vi "Acq-module.vi"(7 "IntermediateFIFO":refnum<k21>="FIFO0", 8 "NumChannels":T1, 9 "SamplingRate0":u16=10000, 11 "Cluster in":T3) -> (3 "cluster out":T4)   [LabVIEW 2013]
uses:
  ctl.ctl
  N Channels.ctl
  <vilib>/rvi/DataTransferAndStorage/Container/Common/niFpgaContainerExecOnDevCompGetState.vi
  <vilib>/rvi/FIFO/Fifo_Resource/nirvififoEmulationWriteFpgaImpl.vi
  <vilib>/rvi/DataTransferAndStorage/Container/Common/niFpgaContainerGetUniqueNameForEmu.vi
  <vilib>/rvi/interface/RandomDataEmulation/nirviRandomDataFPGAFIFO.vi
  <vilib>/rvi/interface/RandomDataEmulation/niFpgaRandomDataHandleErrors.vi
  <vilib>/rvi/eio/common/nirviEmuReportErrorAndStop.vi
  GlobalReg.vi
  <vilib>/rvi/DataTransferAndStorage/Container/XNode/niFpgaContainer.xnode
  <vilib>/rvi/FIFO/Fifo_Resource/niFpgaFifoEmulationRefIn.vi
panel:
  out "Analog Out Cluster":T2
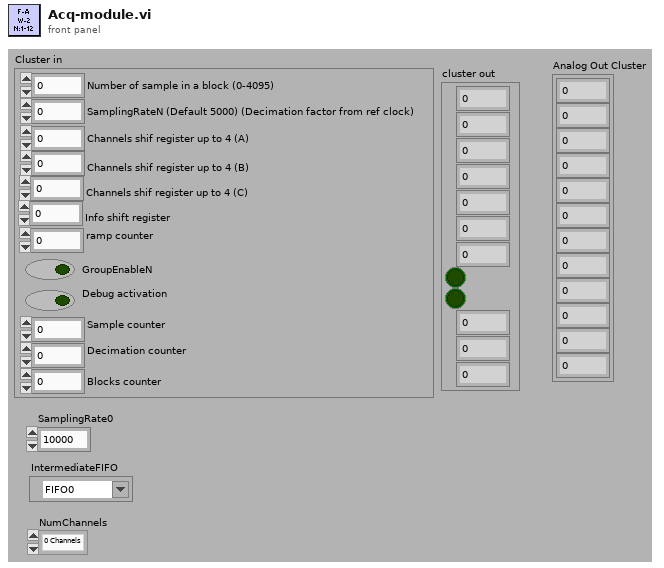
[diagram p1: front panel]
types:
  T1 = typedef "N Channels.ctl" = enum16{"0 Channels", "1 Channels", "2 Channels", "3 Channels", "4 Channels", "5 Channels", "6 Channels", "7 Channels", "8 Channels", "9 Channels", "10 Channels", "11 Channels", "12 Channels"}
  T2 = cluster{i16, i16, i16, i16, i16, i16, i16, i16, i16, i16, i16, i16}
  T3 = typedef "ctl.ctl" = cluster{"Number of sample in a block (0-4095)":u16, "SamplingRateN (Default 5000) (Decimation factor from ref clock)":u16, "Channels shif register up to 4 (A) ":u64, "Channels shif register up to 4 (B) ":u64, "Channels shif register up to 4 (C) ":u64, "Info shift register":u64, "ramp counter":i16, "GroupEnableN":bool, "Debug activation":bool, "Sample counter ":u64, "Decimation counter":u16, "Blocks counter":u16}
  T4 = cluster{u16, u16, u64, u64, u64, u64, i16, bool, bool, u64, u16, u16}
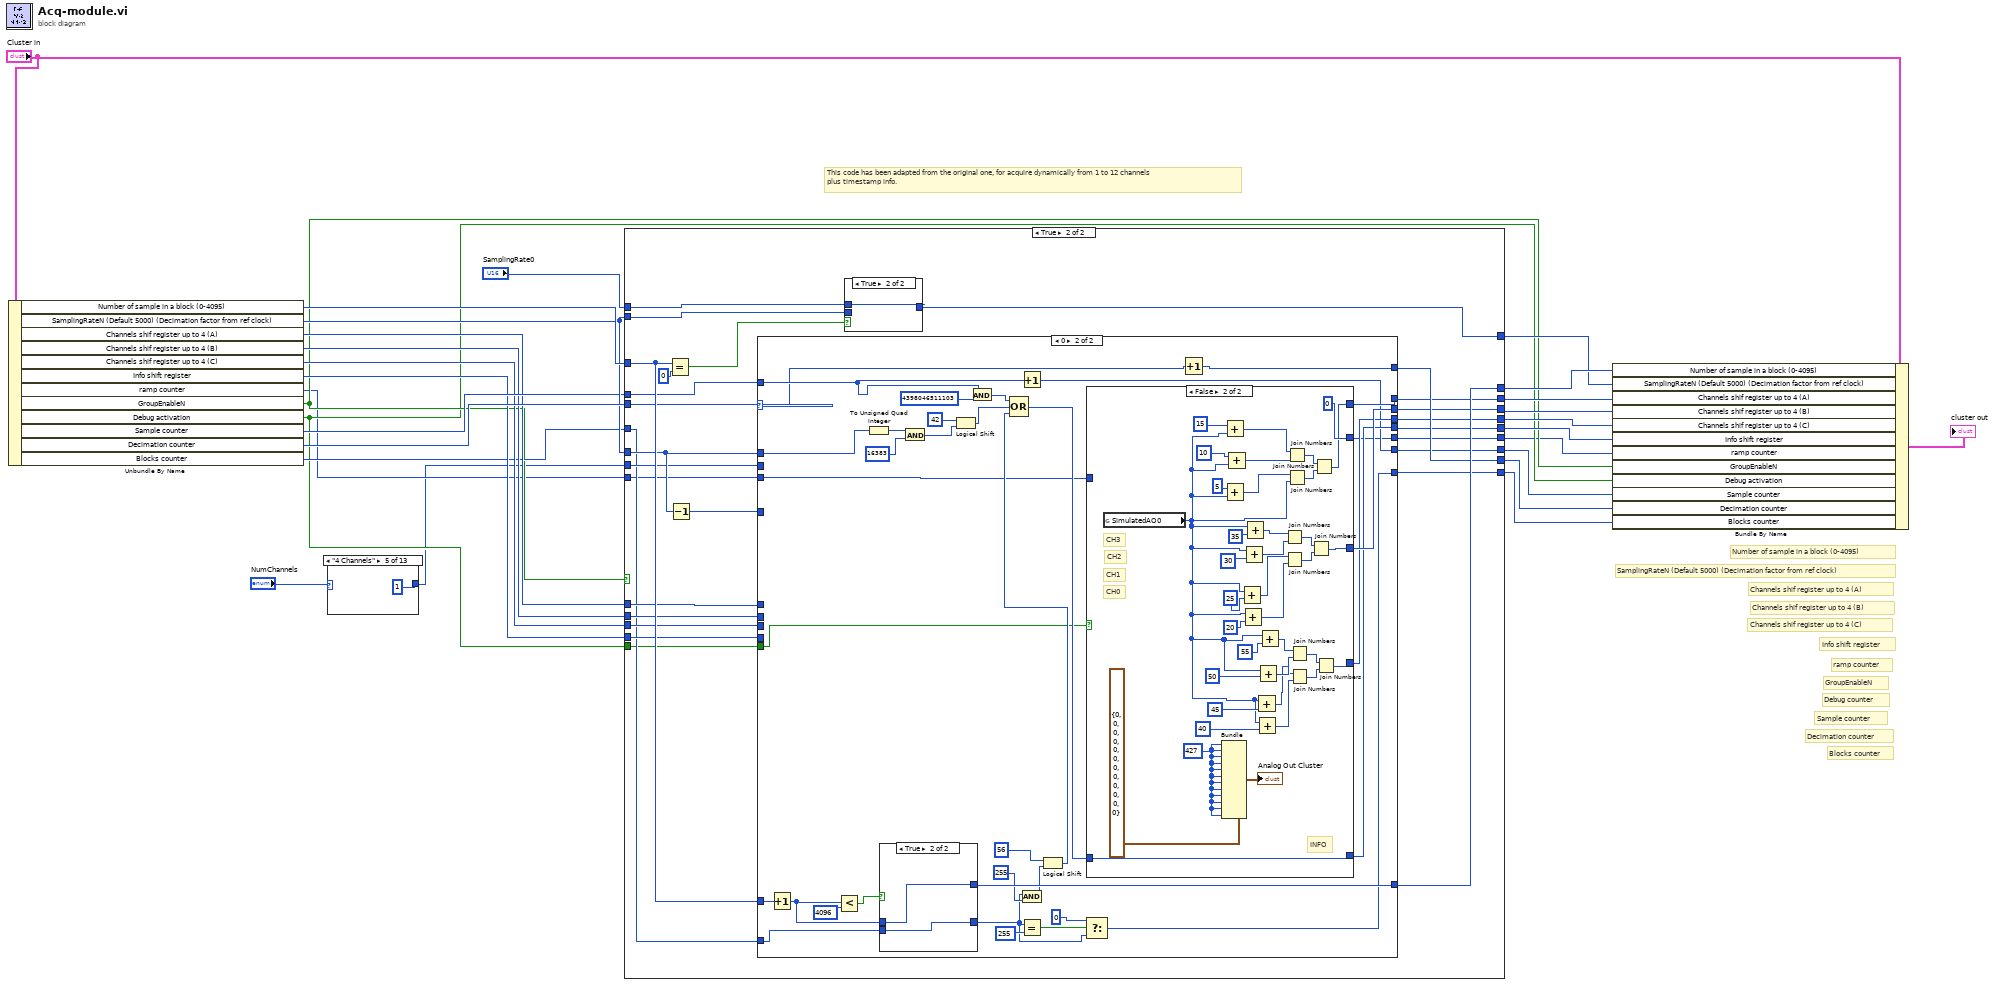
[diagram p0: block diagram]
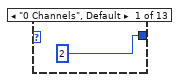
[diagram p2: hidden frame]
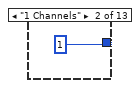
[diagram p3: hidden frame]
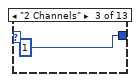
[diagram p4: hidden frame]
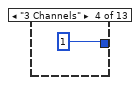
[diagram p5: hidden frame]
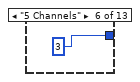
[diagram p6: hidden frame]
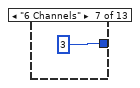
[diagram p7: hidden frame]
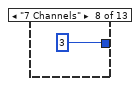
[diagram p8: hidden frame]
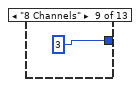
[diagram p9: hidden frame]
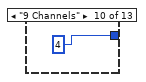
[diagram p10: hidden frame]
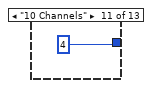
[diagram p11: hidden frame]
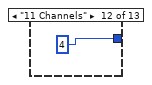
[diagram p12: hidden frame]
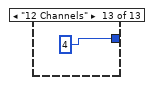
[diagram p13: hidden frame]
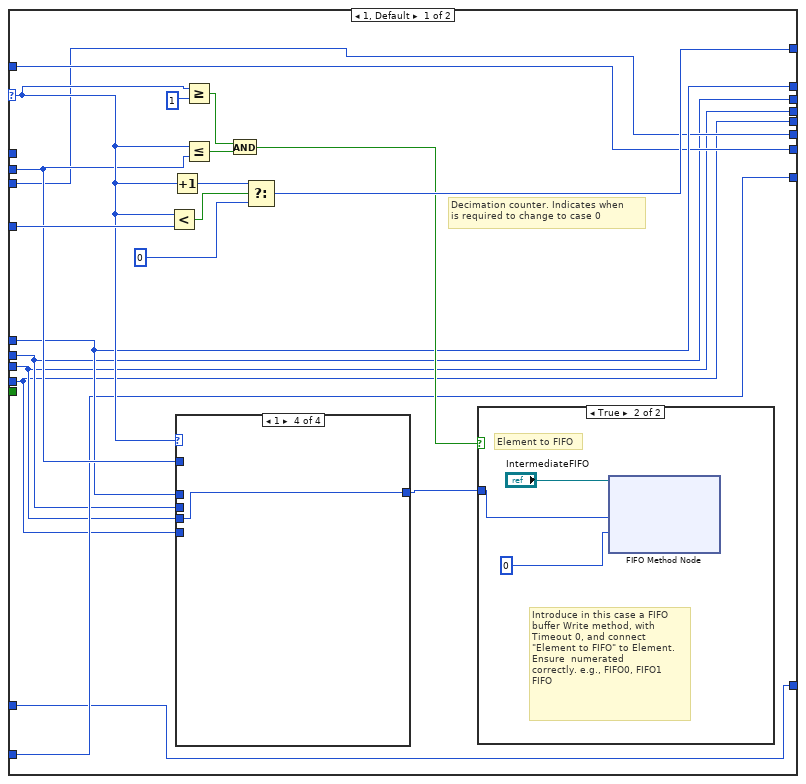
[diagram p15: hidden frame]
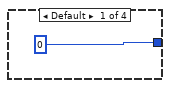
[diagram p17: hidden frame]
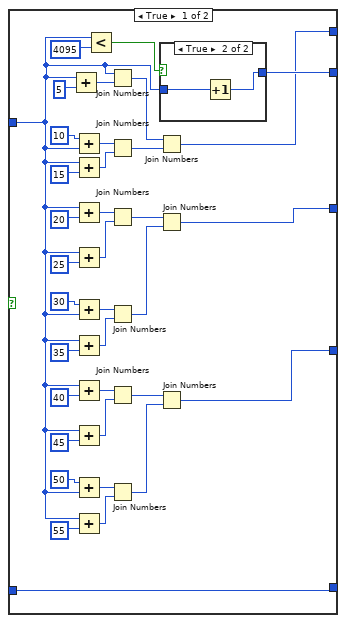
[diagram p20: hidden frame]
diagram:
  # "This code has been adapted from the original one, for acquire dynamically from 1 to 12 channels\nplus timestamp info."
  # "Blocks counter"
  # "Decimation counter"
  # "Sample counter"
  # "Debug counter"
  # "ramp counter"
  # "Info shift register"
  # "Channels shif register up to 4 (C)"
  # "Channels shif register up to 4 (B)"
  # "Channels shif register up to 4 (A)"
  # "SamplingRateN (Default 5000) (Decimation factor from ref clock)"
  # "Number of sample in a block (0-4095)"
  # "GroupEnableN"
  n1 = Unbundle By Name("Cluster in") -> ("Number of sample in a block (0-4095)"=w27:u16, "SamplingRateN (Default 5000) (Decimation factor from ref clock)"=w18:u16, "Channels shif register up to 4 (A)"=w15:u64, "Channels shif register up to 4 (B)"=w14:u64, "Channels shif register up to 4 (C)"=w13:u64, "Info shift register"=w12:u64, "ramp counter"=w7:i16, "GroupEnableN"=w9:bool, "Debug activation"=w8:bool, "Sample counter"=w17:u64, "Decimation counter"=w24:u16, "Blocks counter"=w11:u16)
  n2 = case shown="\"4 Channels\"" "NumChannels" {
    tunnel: [u8 2 ("Number of words") u8 1 ("Number of words") u8 1 ("Number of words") u8 1 ("Number of words") u8 1 ("Number of words") u8 3 ("Number of words") u8 3 ("Number of words") u8 3 ("Number of words") u8 3 ("Number of words") u8 4 ("Number of words") u8 4 ("Number of words") u8 4 ("Number of words") u8 4 ("Number of words")] -> w5
    frame "0 Channels", Default {
    }
    frame "1 Channels" {
    }
    frame "2 Channels" {
    }
    frame "3 Channels" {
    }
    frame "4 Channels" {
    }
    frame "5 Channels" {
    }
    frame "6 Channels" {
    }
    frame "7 Channels" {
    }
    frame "8 Channels" {
    }
    frame "9 Channels" {
    }
    frame "10 Channels" {
    }
    frame "11 Channels" {
    }
    frame "12 Channels" {
    }
  }
  n3 = case shown="True" w9 {
    tunnel: w27 -> [w48 w73]
    tunnel: "SamplingRate0" -> [_ w76]
    tunnel: w18 -> [w49 w74]
    tunnel: [w48 w72] -> w26
    tunnel: [w49 w71] -> w25
    tunnel: w18 -> [_ w70]
    tunnel: w5 -> [_ w68]
    tunnel: w24 -> [w50 w67]
    tunnel: [w50 w66] -> w23
    tunnel: [w47 w65] -> w22
    tunnel: [w46 w64] -> w21
    tunnel: [w45 w63] -> w20
    tunnel: [w44 w62] -> w19
    tunnel: w17 -> [w43 w61]
    tunnel: [w43 w60] -> w16
    tunnel: w15 -> [w47 w59]
    tunnel: w14 -> [w46 w58]
    tunnel: w13 -> [w45 w57]
    tunnel: w12 -> [w44 w56]
    tunnel: w11 -> [w42 w55]
    tunnel: [w42 w54] -> w10
    tunnel: w8 -> [_ w53]
    tunnel: w7 -> [w41 w52]
    tunnel: [w41 w51] -> w6
    frame False {
    }
    frame True {
      n4 = Equal?(x=w73, y=u16 0) -> (x = y?=w75:bool)
      n5 = Decrement(x=w70) -> (x-1=w69:u16)
      n6 = case shown="0" w67 {
        selector: w67 -> [w89 w106]
        tunnel: w73 -> [w82 w139]
        tunnel: [w82 w135] -> w72
        tunnel: w70 -> [_ w132]
        tunnel: w69 -> [w92 _]
        tunnel: w68 -> [w88 _]
        tunnel: [w91 w105] -> w66
        tunnel: [w86 w119] -> w65
        tunnel: [w80 w118] -> w64
        tunnel: [w79 w117] -> w63
        tunnel: [w78 w116] -> w62
        tunnel: w61 -> [w84 w114]
        tunnel: [w84 w113] -> w60
        tunnel: w59 -> [w86 _]
        tunnel: w58 -> [w80 _]
        tunnel: w57 -> [w79 _]
        tunnel: w56 -> [w78 _]
        tunnel: w55 -> [w83 w112]
        tunnel: [w83 w111] -> w54
        tunnel: w53 -> [_ w110]
        tunnel: w52 -> [w81 w109]
        tunnel: [w81 w108] -> w51
        frame 1, Default {
          # "Decimation counter. Indicates when \nis required to change to case 0"
          n7 = Less?(x=w89, y=w92) -> (x < y?=w85:bool)
          n8 = Increment(x=w89) -> (x+1=w97:u16)
          n9 = case shown="1" w89 {
            tunnel: [u64 0 ("Element") w102 w103 w104] -> w90
            tunnel: w86 -> [_ w102 _ _]
            tunnel: w80 -> [_ _ w103 _]
            tunnel: w79 -> [_ _ _ w104]
            tunnel: w78 -> [_ _ _ _]
            tunnel: w88 -> [_ _ _ _]
            frame Default {
            }
            frame 1 {
            }
            frame 2 {
            }
            frame 3 {
            }
          }
          n10 = Greater Or Equal?(x=w89, y=u16 1) -> (x >= y?=w94:bool)
          n11 = Less Or Equal?(x=w89, y=w88) -> (x <= y?=w93:bool)
          n12 = And(x=w94, y=w93) -> (x .and. y?=w87:bool)
          n13 = Select(t=w97, s=w85, f=u16 0) -> (s? t:f=w91:u16)
          n14 = case shown="True" w87 {
            tunnel: w90 -> [_ w100]
            frame False {
            }
            frame True {
              # "Element to FIFO"
              # "Introduce in this case a FIFO buffer Write method, with Timeout 0, and connect \"Element to FIFO\" to Element. Ensure  numerated\ncorrectly. e.g., FIFO0, FIFO1 \nFIFO"
              n15 = xnode ("FIFO Method Node")("Element"=w100, "Timeout"=0, "FIFO In"="IntermediateFIFO") -> ()  [unwired: 2 out]
            }
          }
        }
        frame 0 {
          n16 = Increment(x=w139) -> (x+1=w136:u16)
          n17 = Less?(x=w136, y=u16 4096) -> (x < y?=w137:bool)
          n18 = To Unsigned Quad Integer(1:w132) -> (0:w134:u64)
          n19 = case shown="True" w137 {
            tunnel: w136 -> [_ w220]
            tunnel: [u16 0 w220] -> w135
            tunnel: w112 -> [w217 w219]
            tunnel: [w216 w219] -> w107
            frame False {
              n20 = Increment(x=w217) -> (x+1=w216:u16)
            }
            frame True {
            }
          }
          n21 = And(x=w134, y=i16 16383) -> (x .and. y?=w131:u64)
          n22 = Logical Shift(y=i8 42, x=w131) -> (x << y=w127:u64)
          n23 = And(x=w114, y=u64 4398046511103) -> (x .and. y?=w128:u64)
          n24 = Increment(x=w114) -> (x+1=w113:u64)
          n25 = And(x=w107, y=u64 255) -> (x .and. y?=w125:u64)
          n26 = Equal?(x=w107, y=u16 255) -> (x = y?=w122:bool)
          n27 = Logical Shift(y=i8 56, x=w125) -> (x << y=w120:u64)
          n28 = Compound Arithmetic op=OR(w128, w127, w120) -> (w115:u64)
          n29 = Select(t=u16 0, s=w122, f=w107) -> (s? t:f=w111:u16)
          n30 = case shown="False" w110 {
            tunnel: [w143 w208] -> w119
            tunnel: [w142 w205] -> w118
            tunnel: [w141 w202] -> w117
            tunnel: [w140 w215] -> w116
            tunnel: w115 -> [w140 w215]
            tunnel: w109 -> [w145 _]
            tunnel: [w144 i16 0] -> w108
            frame True {
              n31 = Add(x=w145, y=i16 5) -> (x+y=w172:i16)
              n32 = Add(x=i16 10, y=w145) -> (x+y=w170:i16)
              n33 = Add(x=w145, y=i16 15) -> (x+y=w168:i16)
              n34 = Add(x=w145, y=i16 20) -> (x+y=w157:i16)
              n35 = Add(x=w145, y=i16 25) -> (x+y=w162:i16)
              n36 = Add(x=i16 30, y=w145) -> (x+y=w160:i16)
              n37 = Add(x=w145, y=i16 35) -> (x+y=w158:i16)
              n38 = Add(x=w145, y=i16 40) -> (x+y=w147:i16)
              n39 = Add(x=w145, y=i16 45) -> (x+y=w152:i16)
              n40 = Add(x=i16 50, y=w145) -> (x+y=w150:i16)
              n41 = Add(x=w145, y=i16 55) -> (x+y=w148:i16)
              n42 = Less?(x=w145, y=i16 4095) -> (x < y?=w166:bool)
              n43 = Join Numbers(hi=w145, lo=w172) -> ((hi.lo)=w175:u32)
              n44 = Join Numbers(hi=w170, lo=w168) -> ((hi.lo)=w174:u32)
              n45 = Join Numbers(hi=w157, lo=w162) -> ((hi.lo)=w165:u32)
              n46 = Join Numbers(hi=w160, lo=w158) -> ((hi.lo)=w164:u32)
              n47 = Join Numbers(hi=w147, lo=w152) -> ((hi.lo)=w155:u32)
              n48 = Join Numbers(hi=w150, lo=w148) -> ((hi.lo)=w154:u32)
              n49 = Join Numbers(hi=w175, lo=w174) -> ((hi.lo)=w143:u64)
              n50 = Join Numbers(hi=w165, lo=w164) -> ((hi.lo)=w142:u64)
              n51 = Join Numbers(hi=w155, lo=w154) -> ((hi.lo)=w141:u64)
              n52 = case shown="True" w166 {
                tunnel: w145 -> [_ w178]
                tunnel: [i16 0 w177] -> w144
                frame False {
                }
                frame True {
                  n53 = Increment(x=w178) -> (x+1=w177:i16)
                }
              }
            }
            frame False {
              w212 = i16 427
              # "CH0"
              # "CH1"
              # "CH2"
              # "CH3"
              # "INFO"
              n54 = global read "GlobalReg.vi" "SimulatedAO0"() -> (w179:i16)
              n55 = Bundle(cluster=T2 {0, 0, 0, 0, 0, 0, 0, 0, 0, 0, 0, 0} ("Cluster 2"), w212, w212, w212, w212, w212, w212, w212, w212, w212, w212, w212, w212) -> (→"Analog Out Cluster":T2)
              n56 = Add(x=i16 15, y=w179) -> (x+y=w197:i16)
              n57 = Add(x=i16 5, y=w179) -> (x+y=w200:i16)
              n58 = Add(x=i16 10, y=w179) -> (x+y=w199:i16)
              n59 = Add(x=w179, y=i16 25) -> (x+y=w189:i16)
              n60 = Add(x=w179, y=i16 20) -> (x+y=w188:i16)
              n61 = Add(x=w179, y=i16 30) -> (x+y=w192:i16)
              n62 = Add(x=w179, y=i16 35) -> (x+y=w193:i16)
              n63 = Add(x=w179, y=i16 45) -> (x+y=w182:i16)
              n64 = Add(x=w179, y=i16 40) -> (x+y=w181:i16)
              n65 = Add(x=w179, y=i16 50) -> (x+y=w183:i16)
              n66 = Add(x=w179, y=i16 55) -> (x+y=w187:i16)
              n67 = Join Numbers(hi=w193, lo=w192) -> ((hi.lo)=w207:u32)
              n68 = Join Numbers(hi=w189, lo=w188) -> ((hi.lo)=w206:u32)
              n69 = Join Numbers(hi=w197, lo=w199) -> ((hi.lo)=w210:u32)
              n70 = Join Numbers(hi=w200, lo=w179) -> ((hi.lo)=w209:u32)
              n71 = Join Numbers(hi=w187, lo=w183) -> ((hi.lo)=w204:u32)
              n72 = Join Numbers(hi=w182, lo=w181) -> ((hi.lo)=w203:u32)
              n73 = Join Numbers(hi=w207, lo=w206) -> ((hi.lo)=w205:u64)
              n74 = Join Numbers(hi=w210, lo=w209) -> ((hi.lo)=w208:u64)
              n75 = Join Numbers(hi=w204, lo=w203) -> ((hi.lo)=w202:u64)
            }
          }
          n76 = Increment(x=w106) -> (x+1=w105:u16)
        }
      }
      n77 = case shown="True" w75 {
        tunnel: w76 -> [_ w222]
        tunnel: [w221 w222] -> w71
        tunnel: w74 -> [w221 _]
        frame False {
        }
        frame True {
        }
      }
    }
  }
  n78 = Bundle By Name(cluster="Cluster in", "Number of sample in a block (0-4095)"=w26, "SamplingRateN (Default 5000) (Decimation factor from ref clock)"=w25, "Channels shif register up to 4 (A)"=w22, "Channels shif register up to 4 (B)"=w21, "Channels shif register up to 4 (C)"=w20, "Info shift register"=w19, "ramp counter"=w6, "GroupEnableN"=w9, "Debug activation"=w8, "Sample counter"=w16, "Decimation counter"=w23, "Blocks counter"=w10) -> (→"cluster out":T3)
